vi "Check Found product.vi"(8 "error in (no error) 5":errorcluster, 10 "Product Name":string, 11 "Module Number  2":dbl=1.0) -> (0 "error out 2":errorcluster, 3 "Found 2":bool)   [LabVIEW 2015, in "Copy of Untitled Library 1.lvlib"]
uses:
  Copy of Untitled Library 1.lvlib
  Controls/Enum Constant.ctl
  <userlib>/origin_lib_main/db_interface/DB Operations Enum.ctl
  <vilib>/addons/database/_DB Variant To Data/Database Variant To Data.xnode
  <userlib>/origin_lib_main/db_interface/DB Interface.lvlib
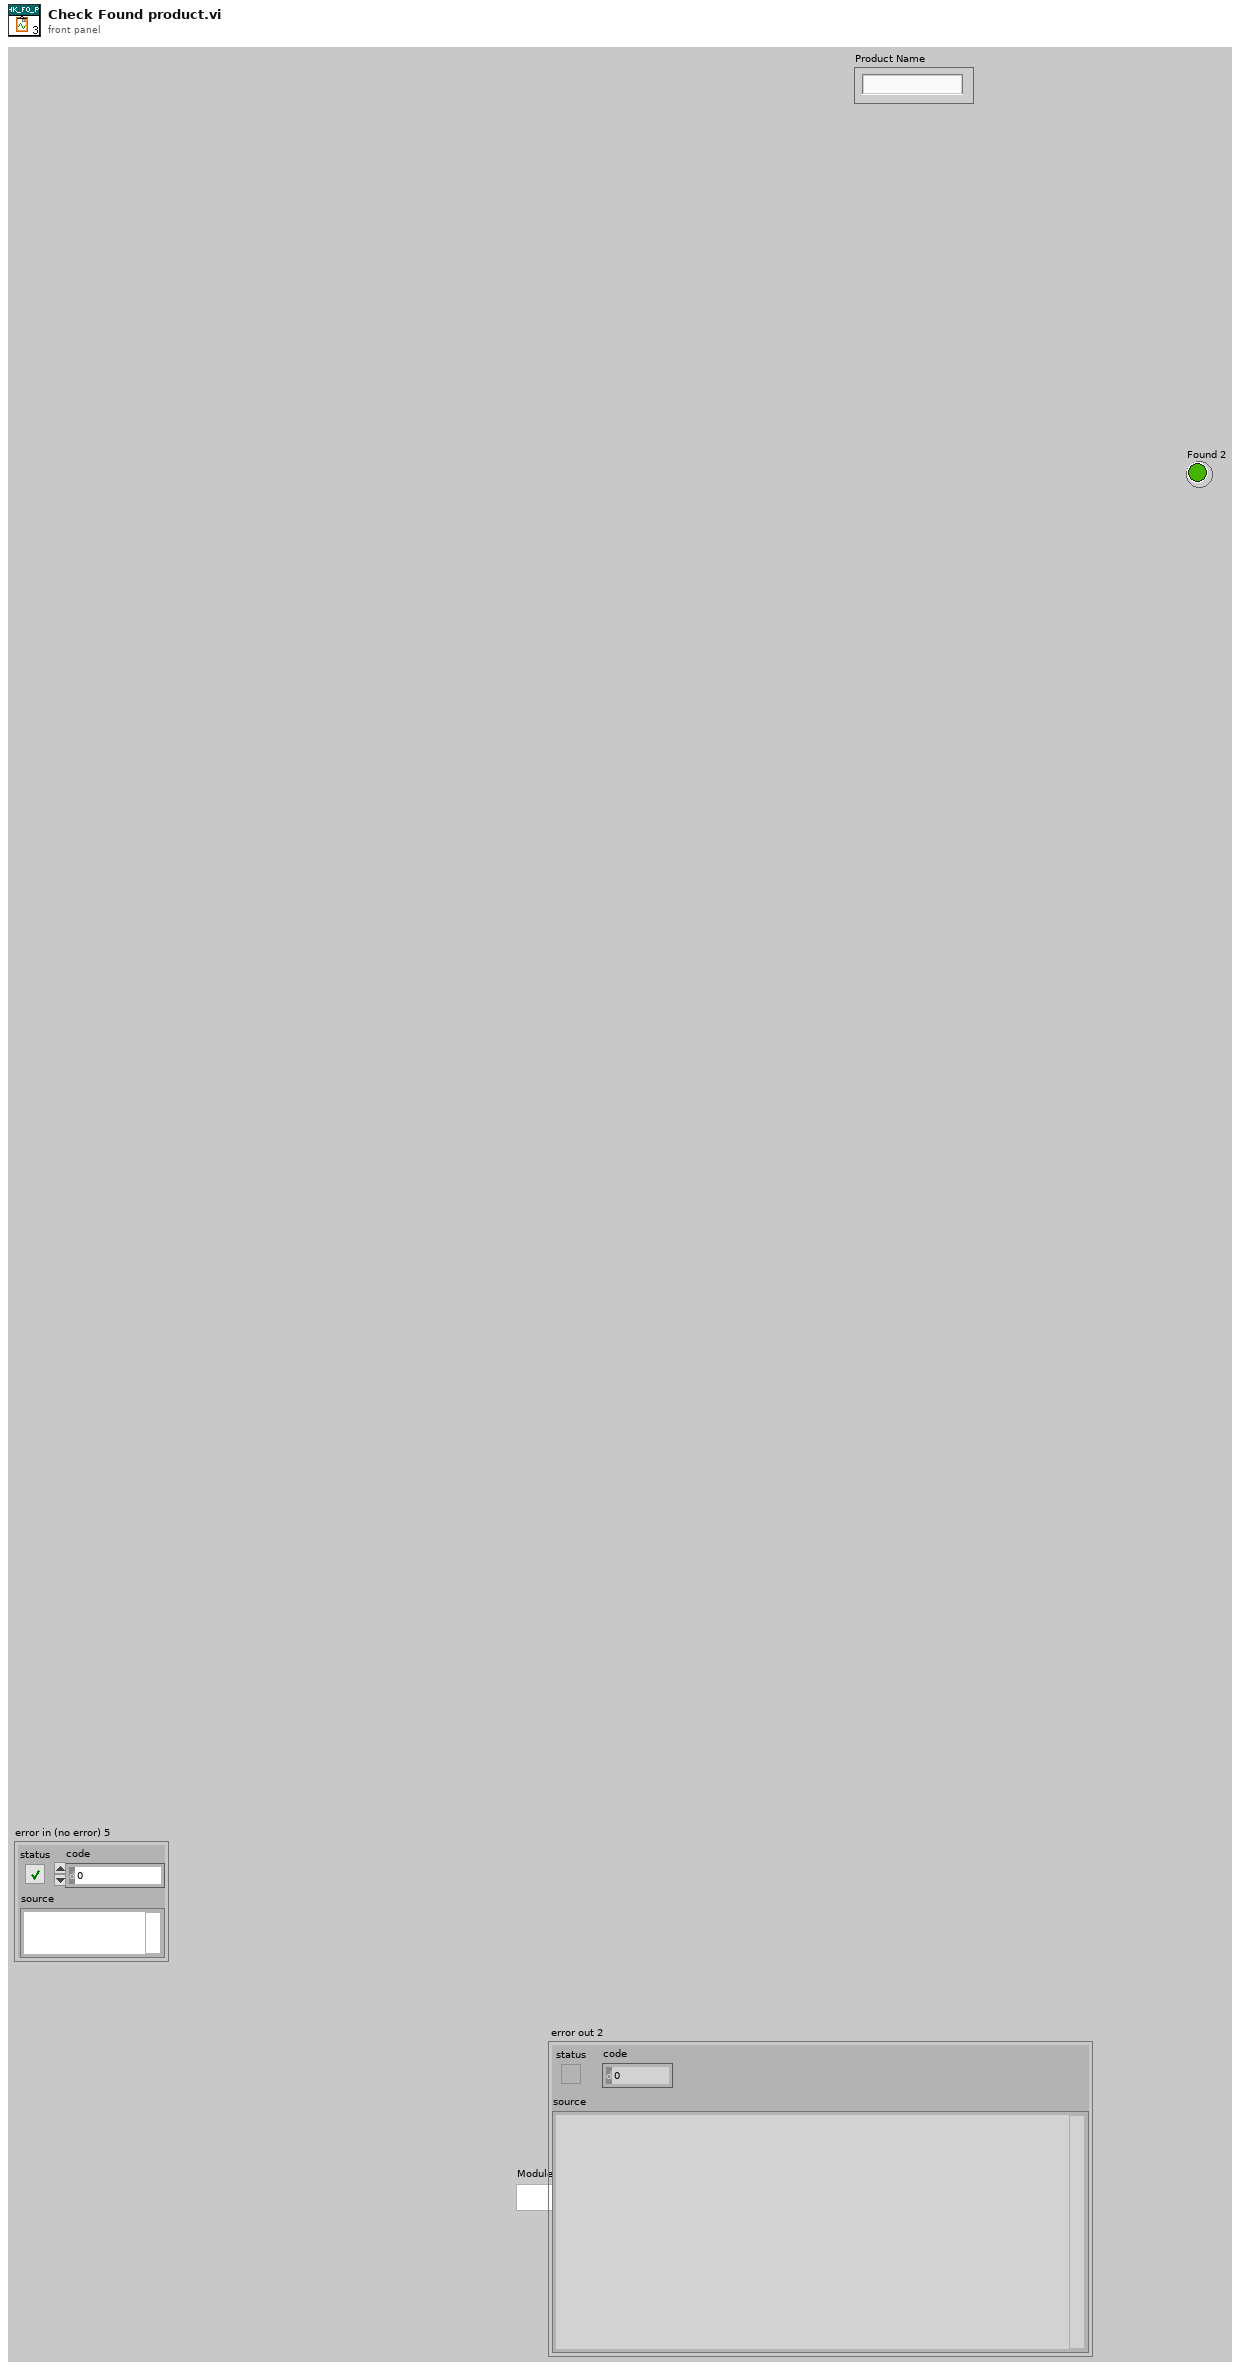
[diagram p1: front panel]
types:
  T1 = typedef "DB Interface.lvlib/DB Operations Enum.ctl" = enum16{"Select", "Update", "Insert", "Delete", "Fetch SQL Query", "Execute SQL Query", "Drop Table", "List Tables"}
  T2 = typedef "Enum Constant.ctl" = enum16{"Init", "Read", "Write"}
  T3 = typedef "FGV Data.ctl" = T4[]
  T4 = typedef "FGV Cluster Data.ctl" = cluster{"Manual/Automatic":bool, "UI Controllers ":string[], "UI Primery Key ":dbl[], "Caller Queue & MSG":T5, "Module ID":dbl, "DB Reference In":T6, "Products Columns":string[], "Cluster":cluster{"Delete Product":enum8{"Enabled", "Disabled", "Disabled and Grayed Out"}, "Add Product ":enum8{"Enabled", "Disabled", "Disabled and Grayed Out"}, "EDIT BATCH":enum8{"Enabled", "Disabled", "Disabled and Grayed Out"}, "Open Batch ":enum8{"Enabled", "Disabled", "Disabled and Grayed Out"}, "Close Batch":enum8{"Enabled", "Disabled", "Disabled and Grayed Out"}, "Delete Batch":enum8{"Enabled", "Disabled", "Disabled and Grayed Out"}, "Add Batch ":enum8{"Enabled", "Disabled", "Disabled and Grayed Out"}}}
  T5 = typedef "Queue and Caller MSG.ctl" = cluster{"Caller Queue":refnum<queue>, "Caller MSG":string}
  T6 = typedef "NI_Database_API.lvlib/Conn ObjectReference.ctl" = refnum<k1>
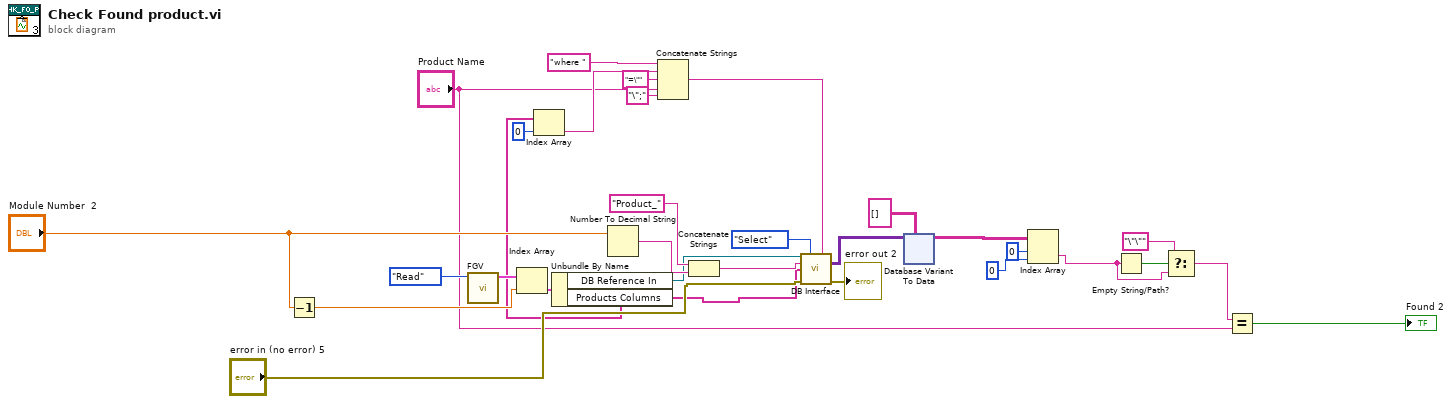
[diagram p0: block diagram]
diagram:
  n1 = Decrement(x="Module Number  2") -> (x-1=w23:dbl)
  n2 = call "FGV.vi"("Enum"=Enum_Constant."Read") -> ("Read Data"=w25:T3)  [unwired: 9 in, 1 out]
  n3 = Index Array(array=w25, index=w23) -> (element=w24:T4)
  n4 = Unbundle By Name(w24) -> ("DB Reference In"=w17:T6, "Products Columns"=w7:string[])
  n5 = Index Array(array=w7, index=0) -> (element=w5:string)
  n6 = Number To Decimal String(number="Module Number  2") -> (decimal integer string=w27:string)  [unwired: 1 in]
  n7 = Concatenate Strings("where " ("string"), w5, "=\"" ("string"), "Product Name", "\";" ("string")) -> (w2:string)
  n8 = Concatenate Strings("Product_" ("string"), w27) -> (w26:string)
  n9 = call <userlib>:"DB Interface.vi"("DB Ref In"=w17, "Operation"=DB_Operations_Enum."Select", "condition"=w2, "DB Table"=w26, "DB columns"=w7, "error in (no error)"="error in (no error) 5") -> ("data Out"=w19:variant[][], "error out"=→"error out 2":errorcluster)  [unwired: 6 in, 2 out]
  n10 = xnode "Database Variant To Data"("database variant"=w19, "type"=string[][] [] ("columns")) -> ("data"=w20:string[][])  [unwired: 1 in, 1 out]
  n11 = Index Array(array=w20, index (row)=0 ("disabled index (row)"), index (col)=0 ("index (row)")) -> (element=w9:string)
  n12 = Empty String/Path?(string/path=w9) -> (empty?=w11:bool)
  n13 = Select(t="\"\"", s=w11, f=w9) -> (s? t:f=w12:string)
  n14 = Equal?(x=w12, y="Product Name") -> (x = y?=→"Found 2":bool)
